vi "Biquadratic peak fit gradient ascent optimisation.vi"(4 "tol^2":dbl=1e-09 format="%#_13g", 5 "Grad step":dbl=0.1 format="%#_13g", 6 "Max iters":i32=10000, 7 "3x3 peak patch":dbl[][](array[numeric])) -> (0 "Iterations":i32, 1 "Sub-pixel convergence":bool, 2 "dy":dbl, 3 "dx":dbl)   [LabVIEW 2014]
uses:
  <vilib>/Analysis/Matrix/Datatypes/RealMatrix.ctl
  <vilib>/Analysis/baseanly.llb/A x Vector.vi
  <vilib>/Analysis/Matrix/NI_Matrix.lvlib
  <vilib>/Analysis/NI_AALBase.lvlib
panel:
  # "Paul Nathan 09/06/2015"
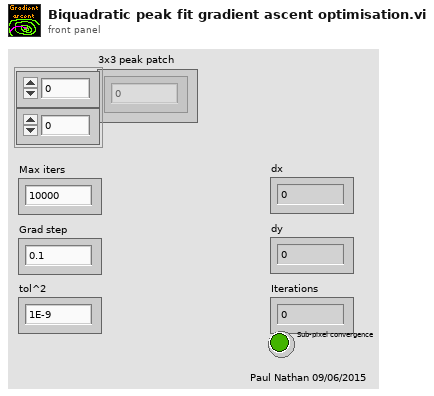
[diagram p1: front panel]
types:
  T1 = typedef "NI_Matrix.lvlib/RealMatrix.ctl" = dbl[][]
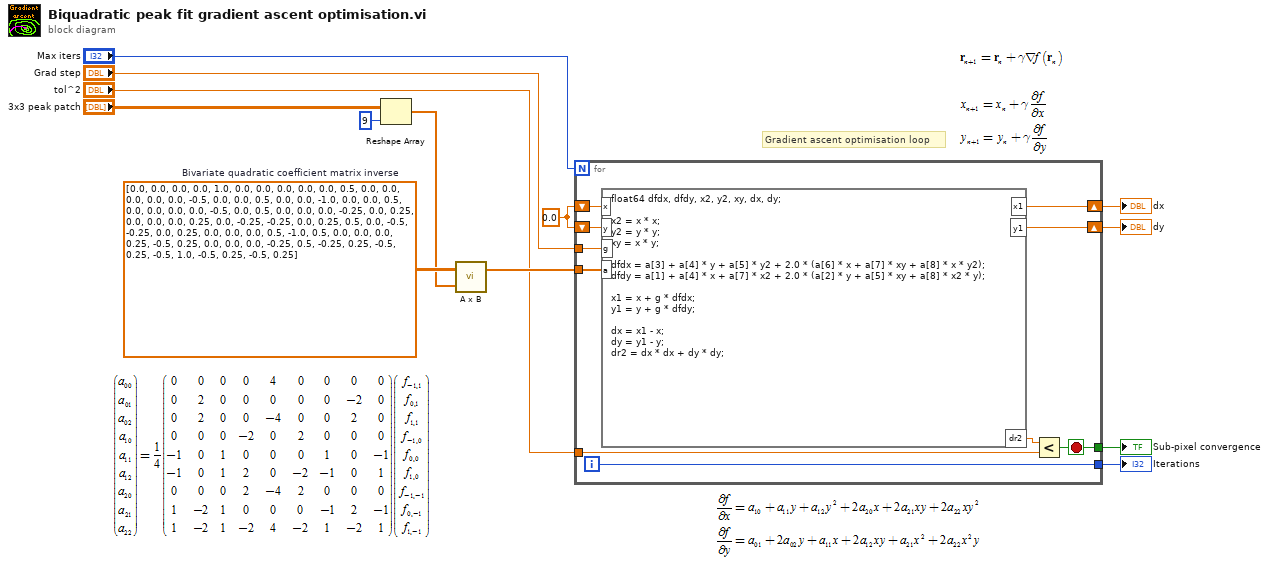
[diagram p0: block diagram]
diagram:
  w10 = 0.0
  w12 = T1 [[0.0, 0.0, 0.0, 0.0, 1.0, 0.0, 0.0, 0.0, 0.0], [0.0, 0.5, 0.0, 0.0, 0.0, 0.0, 0.0, -0.5, 0.0], [0.0, 0.5, 0.0, 0.0, -1.0, 0.0, 0.0, 0.5, 0.0], [0.0, 0.0, 0.0, -0.5, 0.0, 0.5, 0.0, 0.0, 0.0], [-0.25, 0.0, 0.25, 0.0, 0.0, 0.0, 0.25, 0.0, -0.25], [-0.25, 0.0, 0.25, 0.5, 0.0, -0.5, -0.25, 0.0, 0.25], [0.0, 0.0, 0.0, 0.5, -1.0, 0.5, 0.0, 0.0, 0.0], [0.25, -0.5, 0.25, 0.0, 0.0, 0.0, -0.25, 0.5, -0.25], [0.25, -0.5, 0.25, -0.5, 1.0, -0.5, 0.25, -0.5, 0.25]]  # Bivariate quadratic coefficient matrix inverse
  # "Gradient ascent optimisation loop"
  n1 = Reshape Array("3x3 peak patch", 9 ("dimension size")) -> (w11:dbl[])
  n2 = call-poly <vilib>:"A x B.vi"("Vector"=w11, "A"=w12) -> ("A x Vector"=w8:dbl[])  [unwired: 1 out]
  n3 = for {
    N: "Max iters" -> [_]
    shift-right: [w19] -> w2
    shift-left: w10 -> [w20]
    shift-right: [w18] -> w1
    shift-left: w10 -> [w21]
    tunnel: "Grad step" -> [w22]
    tunnel: w8 -> [w23]
    tunnel: "tol^2" -> [w16]
    tunnel: [w15] -> w6
    tunnel: [w14] -> w4
    i -> [w15]
    stop <- w14 stop-if-true
    n4 = formula code="float64 dfdx, dfdy, x2, y2, xy, dx, dy;\n\nx2 = x * x;\ny2 = y * y;\nxy = x * y;\n\ndfdx = a[3] + a[4] * y + a[5] * y2 + 2.0 * (a[6] * x + a[7] * xy + a[8] * x * y2);\ndfdy = a[1] + a[4] * x + a[7] * x2 + 2.0 * (a[2] * y + a[5] * xy + a[8] * x2 * y);\n\nx1 = x + g * dfdx;\ny1 = y + g * dfdy;\n\ndx = x1 - x;\ndy = y1 - y;\ndr2 = dx * dx + dy * dy;"("x"=w20, "y"=w21, "g"=w22, "a"=w23) -> ("x1"=w19:dbl, "y1"=w18:dbl, "dr2"=w17:dbl)
    n5 = Less?(x=w17, y=w16) -> (x < y?=w14:bool)
  }
  "Iterations" <- w6
  "Sub-pixel convergence" <- w4
  "dx" <- w2
  "dy" <- w1
